vi "PH_SHS_Analysis_Statistician.get SHS Analyzer.vi"(0 "i ref in":refnum<vi>, 5 "error in":errorcluster) -> (14 "i ref out":refnum<vi>, 17 "No Analyzer selected?":bool, 19 "error out":errorcluster)   [LabVIEW 2014, in "PH_SHS_Analysis_Statistician.lvlib"]
doc: "This VI queries all Image Operator Instances from the data base. Aterwards it indicates in an GUI which of these instances are running tp allow the user to do a selection."
uses:
  PH_SHS_Analysis_Statistician.lvlib
  CS_Core/CSSystem/CSSystemLib/CSSystemLib.lvlib
  PH_Basics/PH_Common/PH_Common.lvlib
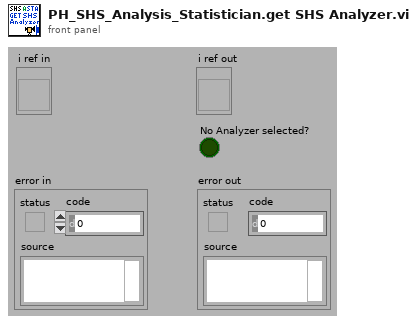
[diagram p1: front panel]
types:
  T1 = typedef "PH_SHS_Analysis_Statistician.lvlib/PH_SHS_Analysis_Statistician.i attribute.ctl" = cluster{"GUI Refs ":cluster{"Status":refnum<vi>, "Result Graph":refnum<vi>, "Mean Data 1":refnum<vi>, "Std Dev Data 1":refnum<vi>, "Mean Data 2":refnum<vi>, "Std Dev Data 2":refnum<vi>, "Mean Data 3":refnum<vi>, "Std Dev Data 3":refnum<vi>, "Dummy Mean":refnum<vi>, "Dummy Std Dev":refnum<vi>, "Export Data":refnum<vi>, "Data 1":refnum<vi>, "Data 2":refnum<vi>, "Data 3":refnum<vi>, "Stat or Trend":refnum<vi>, "Delete":refnum<vi>, "Analyzer":refnum<vi>, "Current Zernike Coefficients":refnum<vi>, "PtV [Lambda]":refnum<vi>, "sample length":refnum<vi>}, "Analyzer":string, "Stat or Trend":bool, "Data 1":i16, "Data 2":i16, "Data 3":i16, "Data":T2[], "sample length":i32, "Datasets strored":i32, "Dataarray Size":i32}
  T2 = typedef "PH_SHS_Analysis.lvlib/PH_SHS_Analysis.Zernike Dataset.ctl" = cluster{"State":T3, "Time Stamp":timestamp, "PtV [lambda]":dbl, "Zernicke Coefficients":T4}
  T3 = typedef "PH_StatusHandler.lvlib/PH_StatusHandler.Status.ctl" = i16
  T4 = typedef "PH_SHS_Analysis.lvlib/PH_SHS_Analysis.Zernike Coefficients.ctl" = cluster{"Tilt x":dbl, "Tilt y":dbl, "Defocus":dbl, "Astig 0°":dbl, "Astig 45°":dbl, "Coma x":dbl, "Coma y":dbl, "Spherical":dbl, "Trefoil 0°":dbl, "Trefoil 30°":dbl, "2nd Astig 0°":dbl, "2nd Astig 45°":dbl, "2nd Coma x":dbl, "2nd Coma y":dbl, "2nd Spherical":dbl}
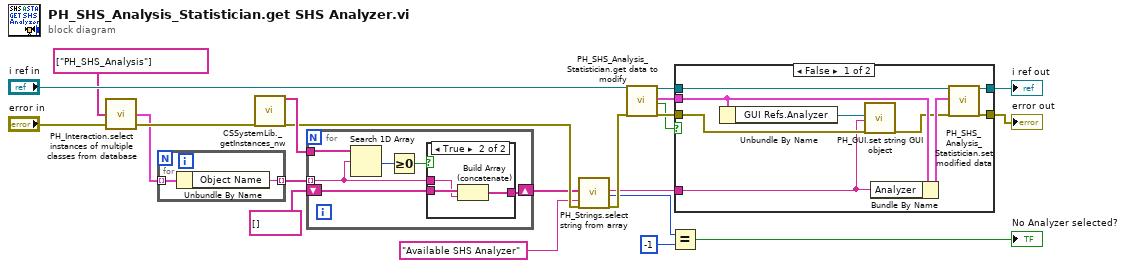
[diagram p0: block diagram]
diagram:
  n1 = call "PH_Interaction.select instances of multiple classes from database.vi"("error in (no error)"="error in", "Classes Input"=string[] ["PH_SHS_Analysis"]) -> ("error out"=w15:errorcluster, "Query Result"=w13:cluster{"Object Name":string, "Class":string}[])  [unwired: 2 in]
  n2 = for {
    tunnel: w13 -> [w24] mode=indexing
    tunnel: [w23] -> w12 mode=indexing
    n3 = Unbundle By Name(w24) -> ("Object Name"=w23:string)
  }
  n4 = call "CSSystemLib._getInstances_nw.vi"("error in (no error)"=w15) -> ("i list"=w17:string[], "error out"=w8:errorcluster)  [unwired: 17 in]
  n5 = for {
    tunnel: w12 -> [w25] mode=indexing
    shift-right: [w29] -> w5
    shift-left: string[] [] ("Query Result") -> [w30]
    tunnel: w17 -> [w26]
    n6 = Search 1D Array(1D array=w26, element=w25) -> (index of element=w27:i32)  [unwired: 1 in]
    n7 = Greater Or Equal To 0?(x=w27) -> (x >= 0?=w28:bool)
    n8 = case shown="True" w28 {
      tunnel: w30 -> [w31 w34]
      tunnel: [w31 w33] -> w29
      tunnel: w25 -> [_ w32]
      frame False {
      }
      frame True {
        n9 = Build Array (concatenate)(w34, w32) -> (w33:string[])
      }
    }
  }
  n10 = call "PH_Strings.select string from array.vi"("String Array in"=w5, "Caption.Text"="Available SHS Analyzer", "error in (no error)"=w8) -> ("string out"=w4:string, "index"=w3:i32, "error out"=w7:errorcluster)  [unwired: 14 in]
  n11 = call "PH_SHS_Analysis_Statistician.get data to modify.vi"("i ref in"="i ref in", "error in (no error)"=w7) -> ("i ref out"=w22:refnum<vi>, "i attribute"=w21:T1, "timed out"=w9:bool, "error out"=w20:errorcluster)  [unwired: 14 in]
  n12 = Equal?(x=w3, y=-1) -> (x = y?=→"No Analyzer selected?":bool)
  n13 = case shown="False" w9 {
    tunnel: w22 -> [w43 w45]
    tunnel: w21 -> [w40 _]
    tunnel: w20 -> [w38 w44]
    tunnel: w4 -> [w35 _]
    tunnel: [w42 w45] -> w11
    tunnel: [w41 w44] -> w10
    frame False {
      n14 = Unbundle By Name(w40) -> ("GUI Refs.Analyzer"=w36:refnum<vi>)
      n15 = call "PH_GUI.set string GUI object.vi"("GUI object Ref"=w36, "Text"=w35, "error in"=w38) -> ("error out"=w37:errorcluster)  [unwired: 16 in]
      n16 = Bundle By Name(cluster=w40, "Analyzer"=w35) -> (w39:T1)
      n17 = call "PH_SHS_Analysis_Statistician.set modified data.vi"("i ref in"=w43, "i attribute"=w39, "error in (no error)"=w37) -> ("i ref out"=w42:refnum<vi>, "error out"=w41:errorcluster)  [unwired: 15 in]
    }
    frame True {
    }
  }
  "i ref out" <- w11
  "error out" <- w10
